vi "Get SwitchOption Info.vi"(8 "error in (no error)":errorcluster, 11 "SwitchOption Msg in":refnum<class "SwitchOption Msg.lvclass">) -> (0 "error out":errorcluster, 1 "ThreadName(\"\")":string, 2 "Base Path":path, 3 "SwitchOption Msg out":refnum<class "SwitchOption Msg.lvclass">, 4 "SubPanelRef":refnum<vi>)   [LabVIEW 2015, in "User_Actor.lvlib" / "SwitchOption Msg.lvclass"]
uses:
  SwitchOption Msg.lvclass
  SwitchOption Msg.lvclass/SwitchOption Msg.ctl
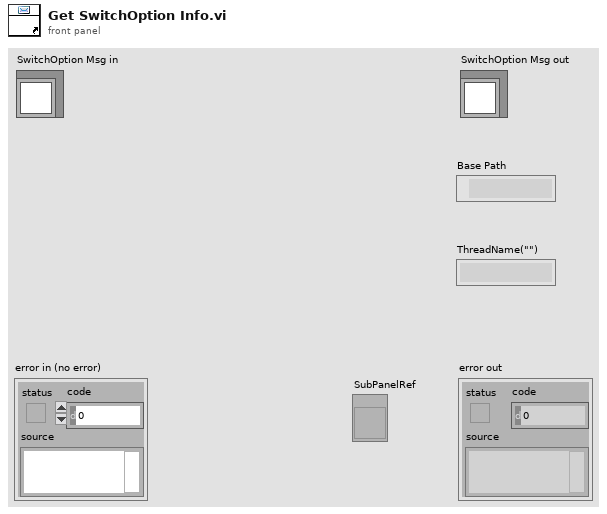
[diagram p1: front panel]
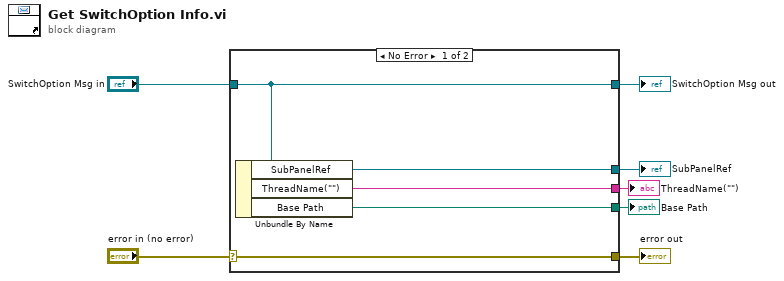
[diagram p0: block diagram]
diagram:
  n1 = case shown="No Error" "error in (no error)" {
    selector: "error in (no error)" -> [w12 w13]
    tunnel: [w12 w13] -> w6
    tunnel: [w11 w14] -> w4
    tunnel: "SwitchOption Msg in" -> [w11 w14]
    tunnel: [w10 _] -> w3
    tunnel: [w9 _] -> w2
    tunnel: [w8 _] -> w1
    frame No Error {
      n2 = Unbundle By Name(w11) -> ("SubPanelRef"=w10:refnum<vi>, "ThreadName(\"\")"=w9:string, "Base Path"=w8:path)
    }
    frame Error {
    }
  }
  "error out" <- w6
  "SwitchOption Msg out" <- w4
  "SubPanelRef" <- w3
  "ThreadName(\"\")" <- w2
  "Base Path" <- w1
